vi "_CallDirectly.vi"() -> ()   [LabVIEW 2019, in "lv-providershell-example2.lvlib"]
uses:
  lv-providershell-example2.lvlib
panel:
  out "Cluster 2":T1
  in  "stop":bool
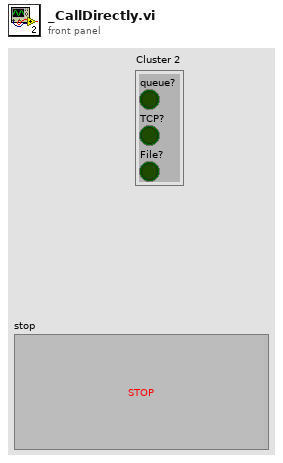
[diagram p1: front panel]
types:
  T1 = cluster{"queue?":bool, "TCP?":bool, "File?":bool}
  T2 = cluster{"queue":refnum<queue>, "TCP":refnum<k5>, "File":refnum<file>}
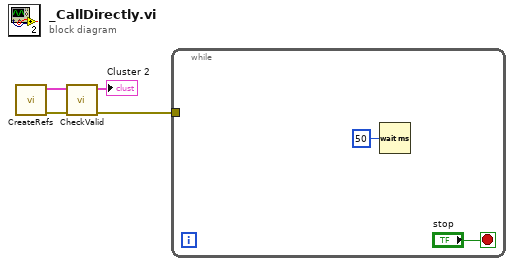
[diagram p0: block diagram]
diagram:
  n1 = call "CreateRefs.vi"() -> ("error out"=w3:errorcluster, "Cluster"=w4:T2)  [unwired: 10 in]
  n2 = call "CheckValid.vi"("error in (no error)"=w3, "Cluster"=w4) -> ("error out"=w2:errorcluster, "Cluster 2"=→"Cluster 2":T1)  [unwired: 8 in]
  n3 = while {
    tunnel: w2 -> [_]
    stop <- "stop" stop-if-true
    n4 = Wait (ms)(milliseconds to wait=u32 50) -> ()  [unwired: 1 out]
  }
